vi "test.vi"(8 "error in (no error)":errorcluster, 11 "BME_DG_Chnl in":refnum<class "BME_DG_Chnl.lvclass">) -> (0 "error out":errorcluster, 3 "BME_DG_Chnl out":refnum<class "BME_DG_Chnl.lvclass">)   [LabVIEW 2009, in "POLARIS BME DG.lvlib" / "BME_DG_Chnl.lvclass"]
uses:
  BME_DG_Chnl.lvclass
  BME_DG_Chnl.lvclass/BME_DG_Chnl.ctl
panel:
  in  "milliseconds to wait 2":u32
  out "ChnlBit":bool
  out "ShotPeriode":dbl
  in  "milliseconds to wait":u32
  in  "stop 2":bool
  in  "stop":bool
  in  "InterruptBits":i32
  in  "Chn Nr":i32
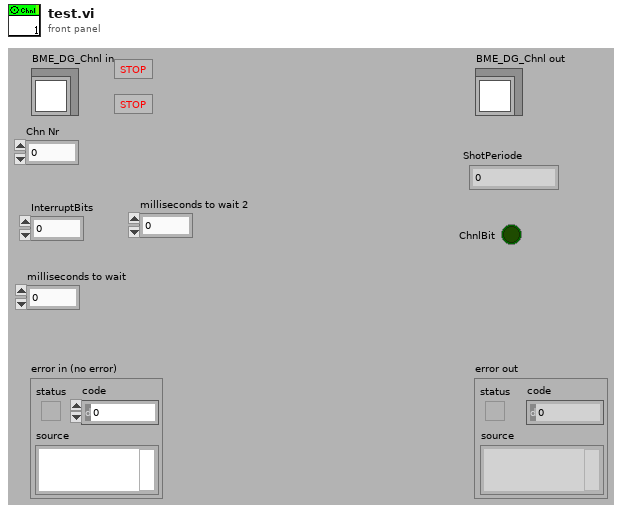
[diagram p1: front panel]
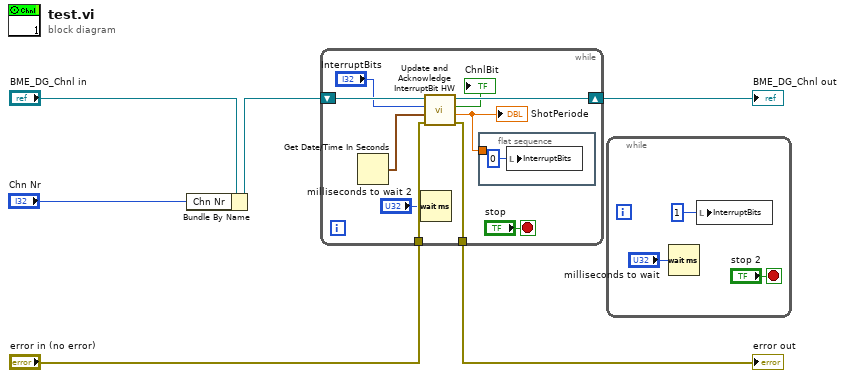
[diagram p0: block diagram]
diagram:
  n1 = Bundle By Name(cluster="BME_DG_Chnl in", "Chn Nr"="Chn Nr") -> (w5:refnum<class "BME_DG_Chnl.lvclass">)
  n2 = while {
    tunnel: "error in (no error)" -> [w15]
    tunnel: [w14] -> w3
    shift-right: [w13] -> w1
    shift-left: w5 -> [w16]
    stop <- "stop" stop-if-true
    n3 = Get Date/Time In Seconds() -> (seconds since 1Jan1904=w8:timestamp)
    n4 = Wait (ms)(milliseconds to wait="milliseconds to wait 2") -> ()  [unwired: 1 out]
    n5 = call "Update and Acknowledge InterruptBit HW.vi"("error in (no error)"=w15, "current time"=w8, "InterruptBits"="InterruptBits", "BME_DG_Chnl in"=w16) -> ("error out"=w14:errorcluster, "ShotPeriode"=w9:dbl, "ChnlBit"=→"ChnlBit":bool, "BME_DG_Chnl out"=w13:refnum<class "BME_DG_Chnl.lvclass">)  [unwired: 4 in]
    "ShotPeriode" <- w9
    n6 = flat-sequence {
      tunnel: w9 -> [_]
      frame #0 {
        n7 = local write "InterruptBits"(0 ("InterruptBits")) -> ()
      }
    }
  }
  "error out" <- w3
  "BME_DG_Chnl out" <- w1
  n8 = while {
    stop <- "stop 2" stop-if-true
    n9 = Wait (ms)(milliseconds to wait="milliseconds to wait") -> ()  [unwired: 1 out]
    n10 = local write "InterruptBits"(1 ("y")) -> ()
  }
